vi "WIPSlowMoving.vi"() -> ()   [LabVIEW 2012]
uses:
  <vilib>/Utility/NIReport.llb/NI_report.lvclass
  <vilib>/addons/database/Connection.llb/DB Tools Open Connec (Path).vi
  <vilib>/addons/database/Connection.llb/Conn Execute.vi
  <vilib>/addons/database/Recordset.llb/Rec Fetch Recordset Data (R).vi
  <vilib>/addons/database/Recordset.llb/Rec Destroy - Connection.vi
  <vilib>/Utility/NIReport.llb/Append Text Table to Report (wrap).vi
  <vilib>/addons/database/_DB Variant To Data/Database Variant To Data.xnode
  <vilib>/addons/database/NI_Database_API.lvlib
  <vilib>/Utility/NIReport.llb/Excel/NI_Excel.lvclass
  <vilib>/addons/_office/NI_ReportGenerationToolkit.lvlib
  <vilib>/Utility/SMTP/NI_SMTPEmail.lvlib
panel:
  in  "Report Template":path=path "O:/Monitor/Report/WIPSlowMoving.xls"
  out "error out 2":errorcluster
  in  "Table Control":string[][](table)
  out "error out 3":errorcluster
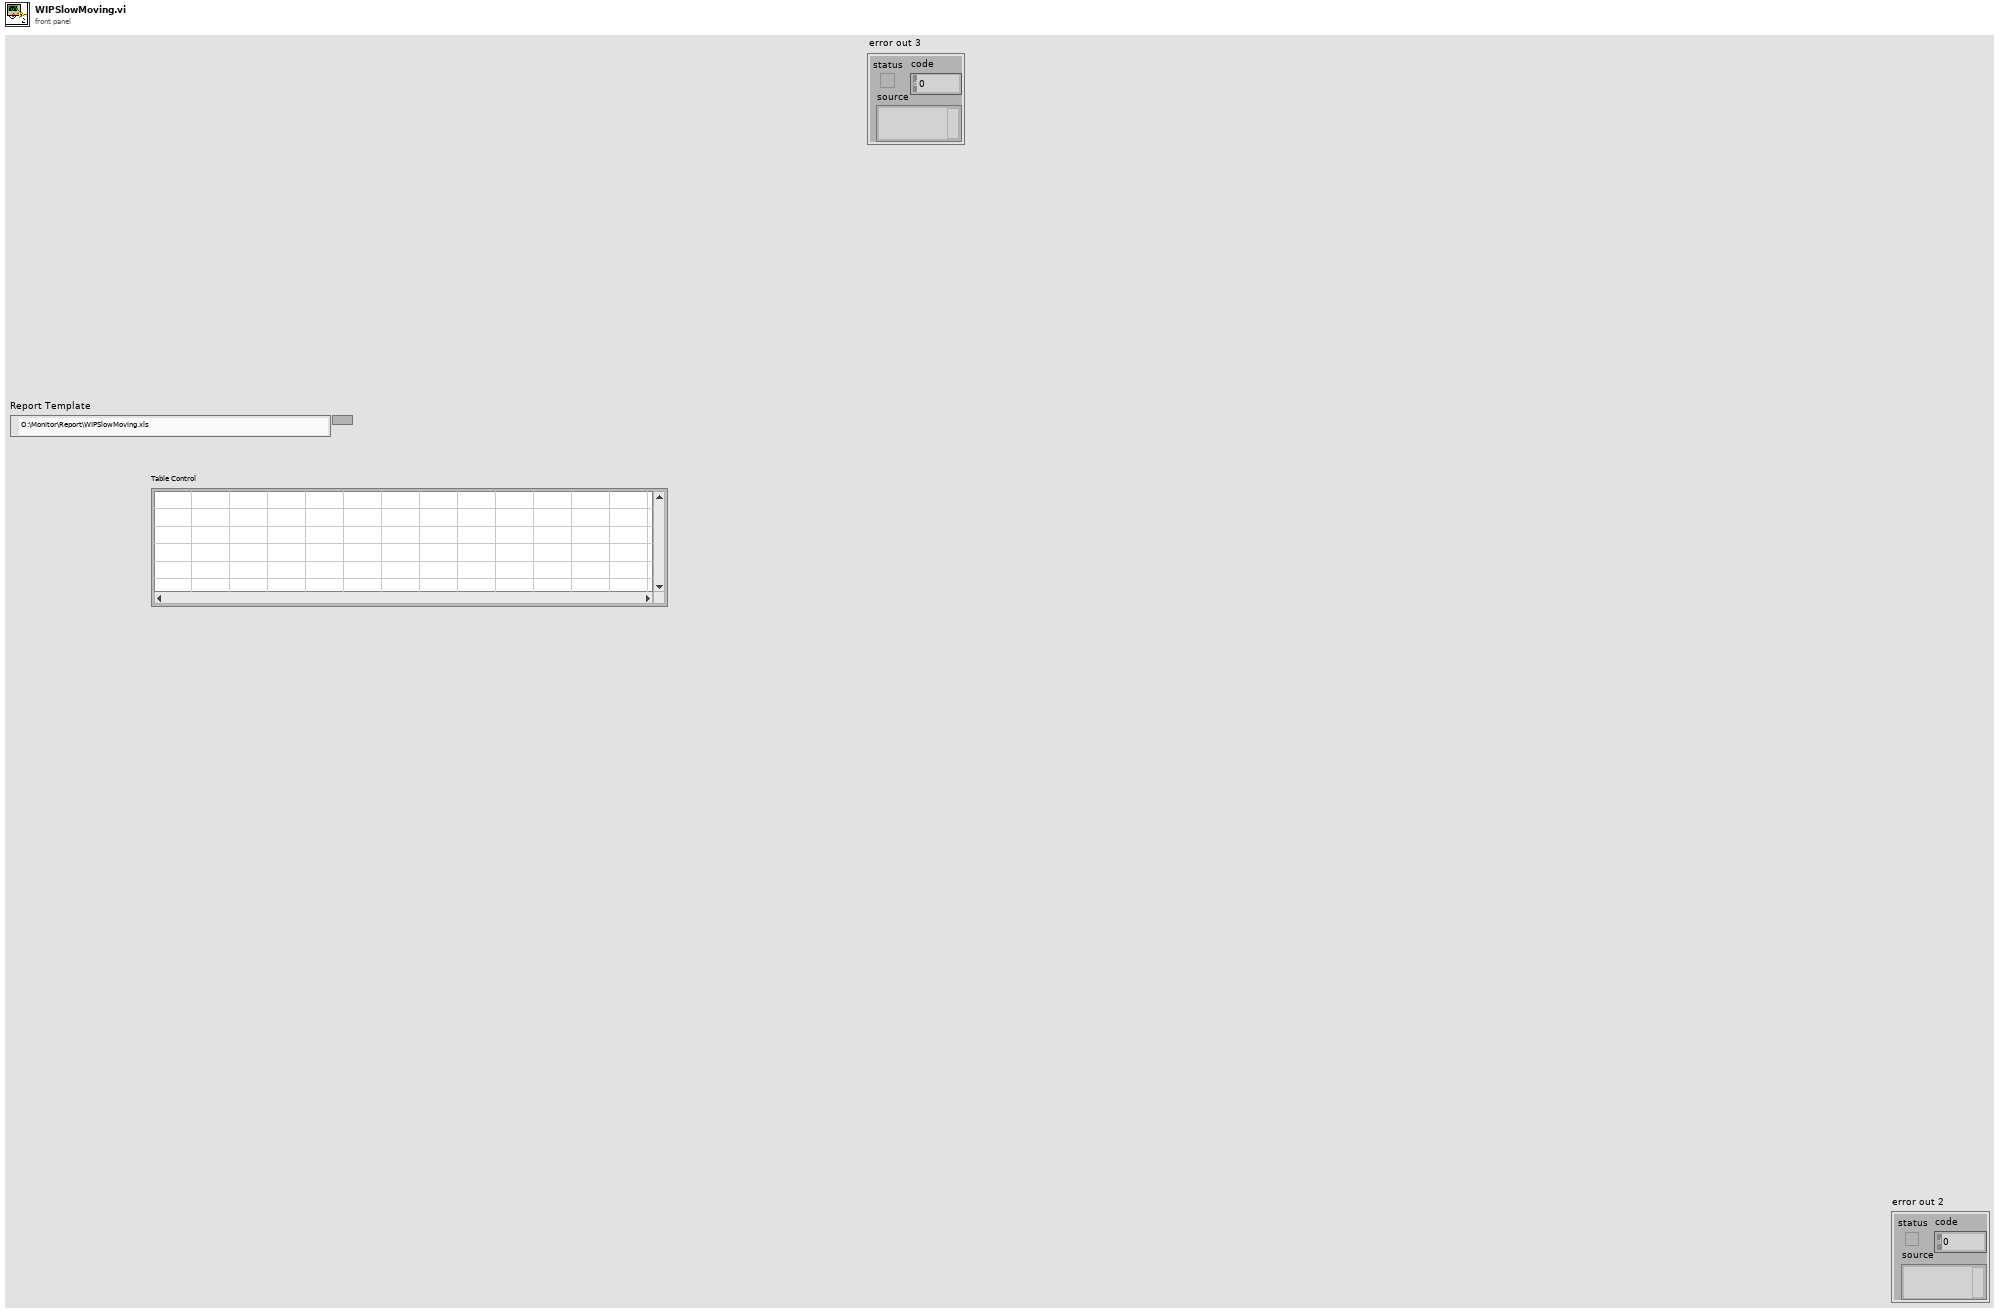
[diagram p1: front panel]
types:
  T1 = typedef "NI_Database_API.lvlib/Conn ObjectReference.ctl" = refnum<k1>
  T2 = typedef "NI_Database_API.lvlib/Rec ObjectReference.ctl" = refnum<k1>
  T3 = enum16{"Standard Report", "HTML", "Word", "Excel"}
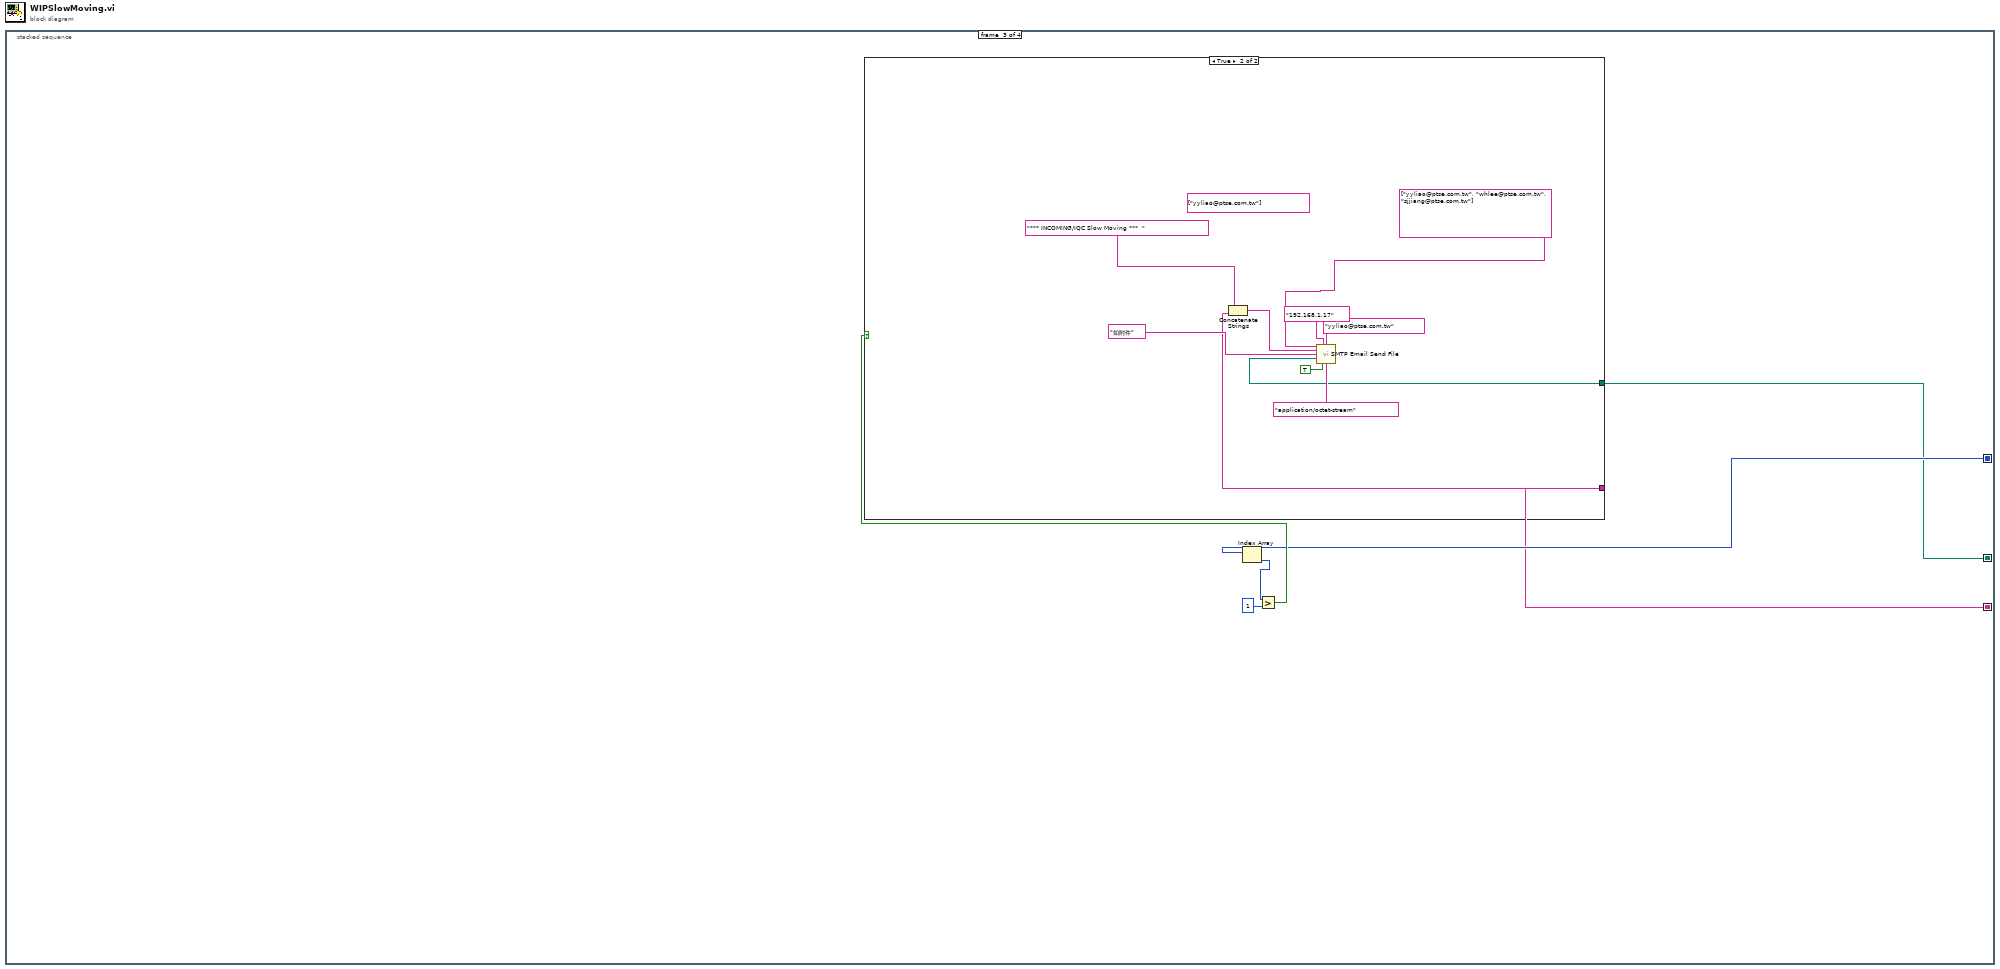
[diagram p0: block diagram]
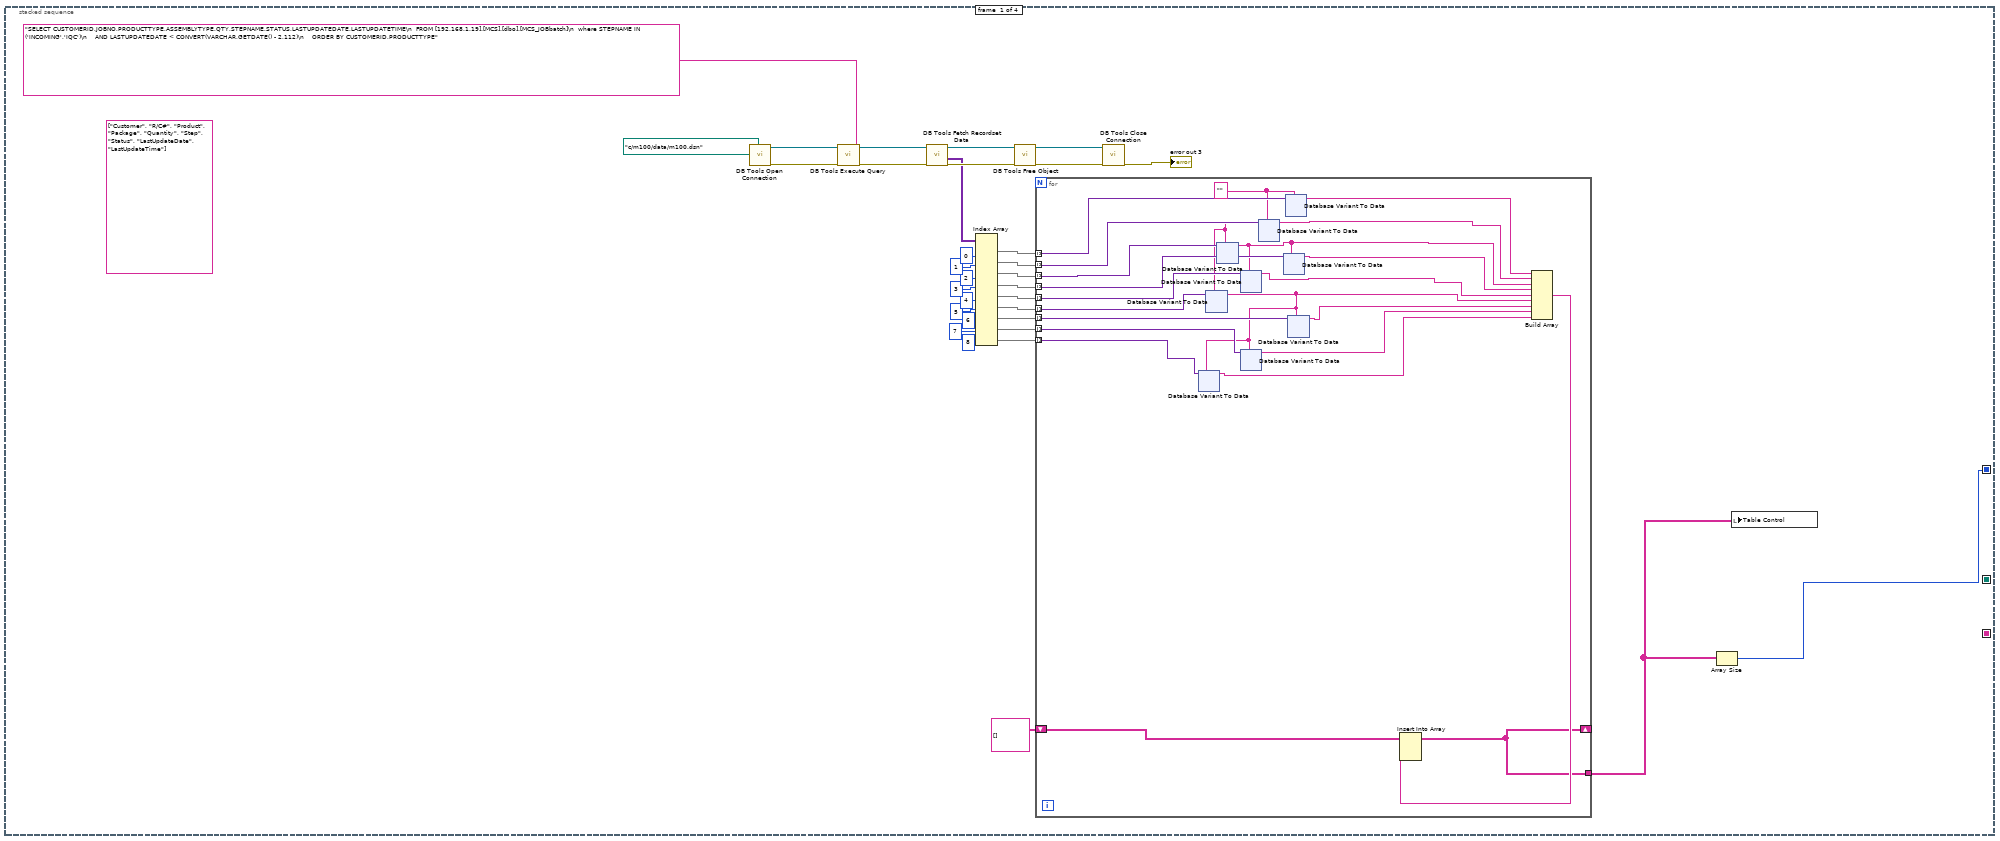
[diagram p2: hidden frame]
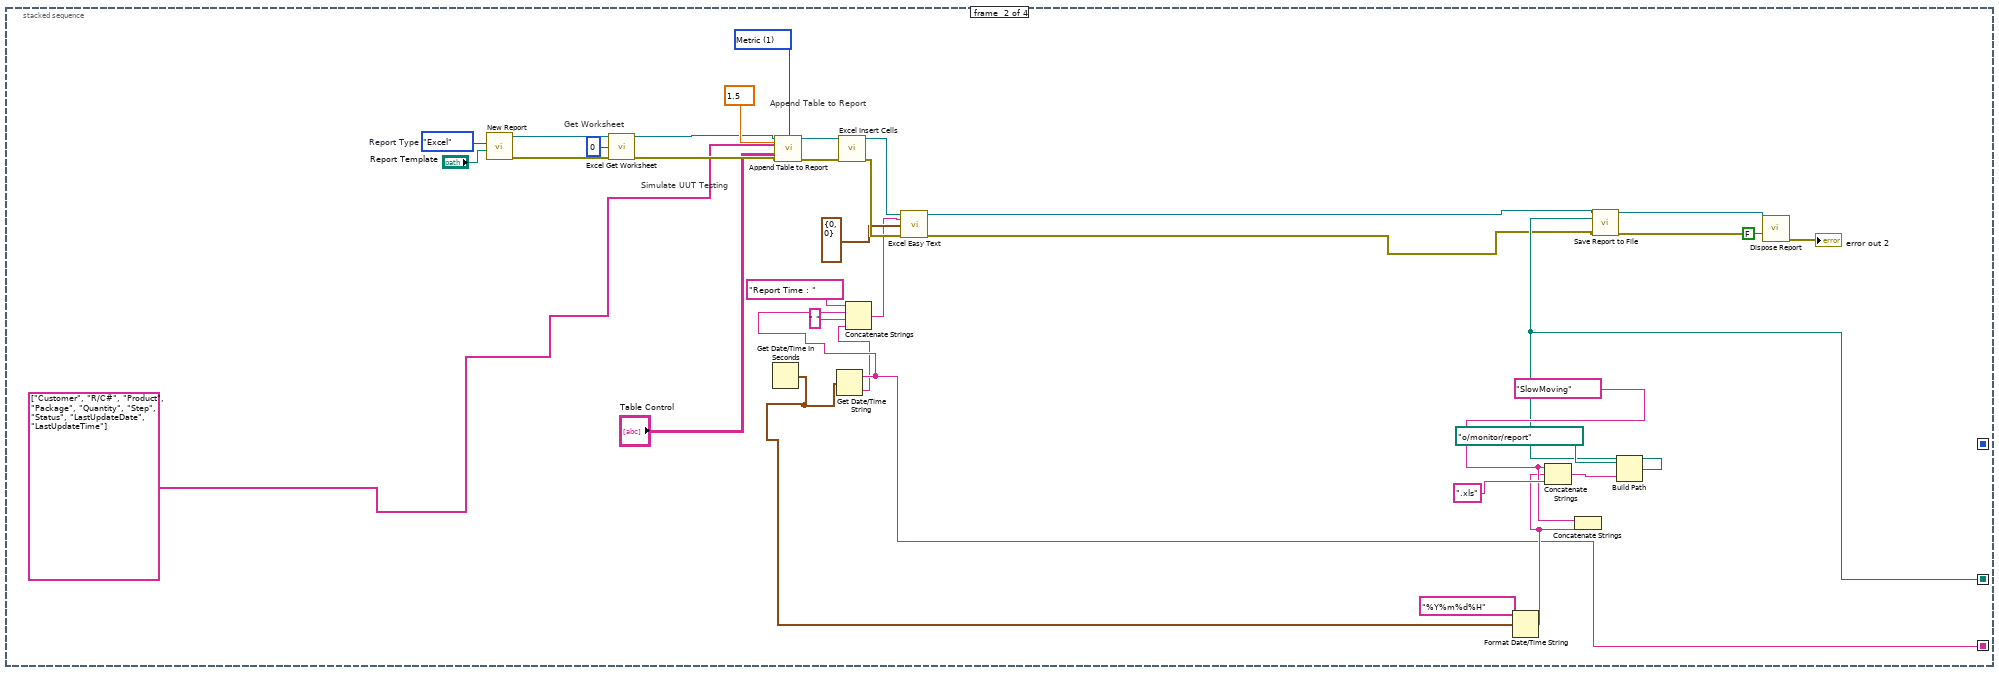
[diagram p3: hidden frame]
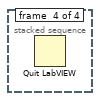
[diagram p5: hidden frame]
diagram:
  n1 = stacked-sequence {
    seq-local: [w1 _ _ _] -> [_ _ w381 _]
    seq-local: [_ w352 _ _] -> [_ _ w380 _]
    seq-local: [_ w349 _ _] -> [_ _ w379 _]
    frame #0 {
      (unwired) string[] ["Customer", "R/C#", "Product", "Package", "Quantity", "Step", "Status", "LastUpdateDate", "LastUpdateTime"] ("row headers")
      n2 = call-poly <vilib>:"DB Tools Open Connection.vi"("connection information"=path "c:/m100/data/m100.dsn") -> ("error out"=w28:errorcluster, "connection reference"=w32:T1)  [unwired: 7 in]
      n3 = call-poly <vilib>:"DB Tools Execute Query.vi"("error in (no error)"=w28, "SQL query"="SELECT CUSTOMERID,JOBNO,PRODUCTTYPE,ASSEMBLYTYPE,QTY,STEPNAME,STATUS,LASTUPDATEDATE,LASTUPDATETIME\n  FROM [192.168.1.19].[MCS].[dbo].[MCS_JOBbatch]\n  where STEPNAME IN ('INCOMING','IQC')\n    AND LASTUPDATEDATE < CONVERT(VARCHAR,GETDATE() - 2,112)\n    ORDER BY CUSTOMERID,PRODUCTTYPE", "connection reference"=w32) -> ("error out"=w27:errorcluster, "recordset reference"=w31:T2)  [unwired: 5 in]
      n4 = call-poly <vilib>:"DB Tools Fetch Recordset Data.vi"("error in (no error)"=w27, "recordset reference"=w31) -> ("error out"=w26:errorcluster, "recordset data"=w10:variant[][], "recordset reference out"=w30:T2)  [unwired: 3 in]
      n5 = Index Array(array=w10, index (col) #1=0 ("disabled index (col)"), index (col) #2=1 ("index (col)"), index (col) #3=2 ("index (col)"), index (col) #4=3 ("index (col)"), index (col) #5=4 ("index (col)"), index (col) #6=5 ("index (col)"), index (col) #7=6 ("index (col)"), index (col) #8=7 ("index (col)"), index (col) #9=8 ("index (col)")) -> (element #1=w17:variant[], element #2=w16:variant[], element #3=w15:variant[], element #4=w14:variant[], element #5=w13:variant[], element #6=w12:variant[], element #7=w5:variant[], element #8=w4:variant[], element #9=w3:variant[])  [unwired: 9 in]
      n6 = call-poly <vilib>:"DB Tools Free Object.vi"("error in (no error)"=w26, "recordset reference"=w30) -> ("error out"=w25:errorcluster, "connection reference"=w29:T1)  [unwired: 8 in]
      n7 = for {
        tunnel: w17 -> [w55] mode=indexing
        tunnel: w16 -> [w54] mode=indexing
        tunnel: w15 -> [w53] mode=indexing
        tunnel: w14 -> [w52] mode=indexing
        tunnel: w13 -> [w51] mode=indexing
        tunnel: w12 -> [w50] mode=indexing
        tunnel: [w47] -> w2
        shift-right: [w47] -> _
        shift-left: string[][] [] -> [w46]
        tunnel: w5 -> [w40] mode=indexing
        tunnel: w4 -> [w39] mode=indexing
        tunnel: w3 -> [w38] mode=indexing
        w43 = ""
        n8 = xnode "Database Variant To Data"("database variant"=w50, "type"=w43) -> ("data"=w36:string)  [unwired: 1 in, 1 out]
        n9 = xnode "Database Variant To Data"("database variant"=w38, "type"=w36) -> ("data"=w34:string)  [unwired: 1 in, 1 out]
        n10 = xnode "Database Variant To Data"("database variant"=w53, "type"=w43) -> ("data"=w42:string)  [unwired: 1 in, 1 out]
        n11 = xnode "Database Variant To Data"("database variant"=w51, "type"=w42) -> ("data"=w41:string)  [unwired: 1 in, 1 out]
        n12 = xnode "Database Variant To Data"("database variant"=w39, "type"=w36) -> ("data"=w35:string)  [unwired: 1 in, 1 out]
        n13 = xnode "Database Variant To Data"("database variant"=w54, "type"=w43) -> ("data"=w45:string)  [unwired: 1 in, 1 out]
        n14 = xnode "Database Variant To Data"("database variant"=w52, "type"=w42) -> ("data"=w44:string)  [unwired: 1 in, 1 out]
        n15 = xnode "Database Variant To Data"("database variant"=w55, "type"=w43) -> ("data"=w49:string)  [unwired: 1 in, 1 out]
        n16 = xnode "Database Variant To Data"("database variant"=w40, "type"=w36) -> ("data"=w37:string)  [unwired: 1 in, 1 out]
        n17 = Build Array(w49, w45, w42, w44, w41, w36, w37, w35, w34) -> (w48:string[])
        n18 = Insert Into Array(array=w46, new element=w48) -> (w47:string[][])  [unwired: 2 in]
      }
      n19 = call <vilib>:"DB Tools Close Connection.vi"("error in (no error)"=w25, "connection reference"=w29) -> ("error out"=→"error out 3":errorcluster)  [unwired: 5 in]
      n20 = Array Size(array=w2) -> (size(s)=w1:i32[])
      n21 = local write "Table Control"(w2) -> ()
    }
    frame #1 {
      w356 = u16 1 items=["US", "Metric", "Default"] ("measurement system")
      w357 = "SlowMoving"
      w378 = T3."Excel"  # Report Type
      # "Simulate UUT Testing"
      # "Append Table to Report"
      # "Get Worksheet"
      n22 = call <vilib>:"New Report.vi"("report type"=w378, "template (empty)"="Report Template") -> ("report out"=w373:refnum<class "NI_report.lvclass">, "error out"=w372:errorcluster)  [unwired: 12 in]
      n23 = call <vilib>:"Excel Get Worksheet.vi"("report in"=w373, "worksheet index (0)"=0, "error in (no error)"=w372) -> ("report out"=w362:refnum<class "NI_report.lvclass">, "error out"=w361:errorcluster)  [unwired: 11 in]
      n24 = Get Date/Time In Seconds() -> (seconds since 1Jan1904=w347:timestamp)
      n25 = call-poly <vilib>:"Append Table to Report.vi"("report in"=w362, "column width (1)"=1.5, "measurement system"=w356, "column headers"=string[] ["Customer", "R/C#", "Product", "Package", "Quantity", "Step", "Status", "LastUpdateDate", "LastUpdateTime"] ("row headers"), "text data"="Table Control", "error in (no error)"=w361) -> ("report out"=w375:refnum<class "NI_report.lvclass">, "error out"=w374:errorcluster)  [unwired: 6 in, 2 out]
      n26 = Get Date/Time String(seconds (now)=w347) -> (date string=w349:string, time string=w348:string)  [unwired: 2 in]
      n27 = call <vilib>:"Excel Insert Cells.vi"("report in"=w375, "error in (no error)"=w374) -> ("report out"=w369:refnum<class "NI_report.lvclass">, "error out"=w368:errorcluster)  [unwired: 12 in]
      n28 = Concatenate Strings("Report Time : " ("string"), w349, " " ("string"), w348) -> (w365:string)
      n29 = call <vilib>:"Excel Easy Text.vi"("report in"=w369, "text"=w365, "start (-1, -1)"=cluster{"row":i32, "column":i32} {"row"=0, "column"=0} ("end (-1, -1)"), "error in (no error)"=w368) -> ("report out"=w346:refnum<class "NI_report.lvclass">, "error out"=w345:errorcluster)  [unwired: 7 in, 3 out]
      n30 = Format Date/Time String(time format string (%c)="%Y%m%d%H", seconds (now)=w347) -> (date/time string=w354:string)  [unwired: 1 in]
      n31 = Concatenate Strings(w357, w354, ".xls" ("string")) -> (w358:string)
      n32 = Concatenate Strings(w357, w354) -> ()  [unwired: 1 out]
      n33 = Build Path(base path=path "o:/monitor/report", name or relative path=w358) -> (appended path=w352:path)
      n34 = call-dynamic "Save Report to File.vi"("report in"=w346, "report file path"=w352, "error in (no error)"=w345) -> ("report out"=w364:refnum<class "NI_report.lvclass">, "error out"=w363:errorcluster)  [unwired: 11 in]
      n35 = call-dynamic "Dispose Report.vi"("report in"=w364, "save changes? (F)"=FALSE, "error in (no error)"=w363) -> ("error out"=→"error out 2":errorcluster)  [unwired: 12 in]
    }
    frame #2 {
      n36 = Index Array(array=w381) -> (element=w384:i32)  [unwired: 1 in]
      n37 = Greater?(x=w384, y=1) -> (0:w382:bool)
      n38 = case shown="True" w382 {
        tunnel: w380 -> [_ w389]
        tunnel: w379 -> [_ w386]
        frame False {
        }
        frame True {
          (unwired) string[] ["yyliao@ptse.com.tw"] ("recipients")
          n39 = Concatenate Strings("*** INCOMING/IQC Slow Moving ***  " ("subject ([No Subject])"), w386) -> (w387:string)
          n40 = call <vilib>:"SMTP Email Send File.vi"("recipients"=string[] ["yyliao@ptse.com.tw", "whlee@ptse.com.tw", "sjjiang@ptse.com.tw"], "mail server"="192.168.1.17", "return address"="yyliao@ptse.com.tw", "subject ([No Subject])"=w387, "message"="如附件", "file path"=w389, "binary? (F)"=TRUE, "MIME content-type (application/octet-stream)"="application/octet-stream") -> ()  [unwired: 6 in, 2 out]
        }
      }
    }
    frame #3 {
      n41 = Quit LabVIEW() -> ()  [unwired: 1 in]
    }
  }
